vi "Is Post Step Runtime Error.vi"(11 "error in":errorcluster) -> (4 "Is Post Step Runtime Error":bool, 15 "error out":errorcluster)   [LabVIEW 2023, in "RFFixtureCharact.Public.lvlib"]
uses:
  RFFixtureCharact.Public.lvlib
  Common/RFCalAndFixtureCharact.Common.lvlib
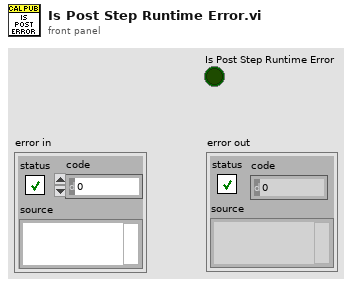
[diagram p1: front panel]
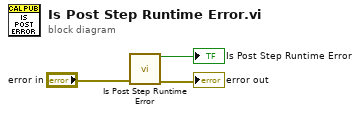
[diagram p0: block diagram]
diagram:
  n1 = call "Is Post Step Runtime Error.vi"("error in"="error in") -> ("Is Post Step Runtime Error"=→"Is Post Step Runtime Error":bool, "error out"=→"error out":errorcluster)  [unwired: 13 in]
